vi "time_acquisition_loop.vi"(7 "Period (s)":dbl caption="周期 (s)" format="%#_13g") -> (0 "t0 (scan)":i64 caption="起始时间 (scan)", 1 "Period (scan)":i64 caption="周期 (scan)", 2 "timestamp output":timestamp caption="时间标识输出")   [LabVIEW 2015]
uses:
  globals/global_monitoring_variables.vi
  globals/global_configuration_options.vi
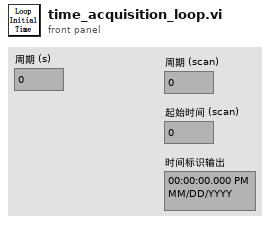
[diagram p1: front panel]
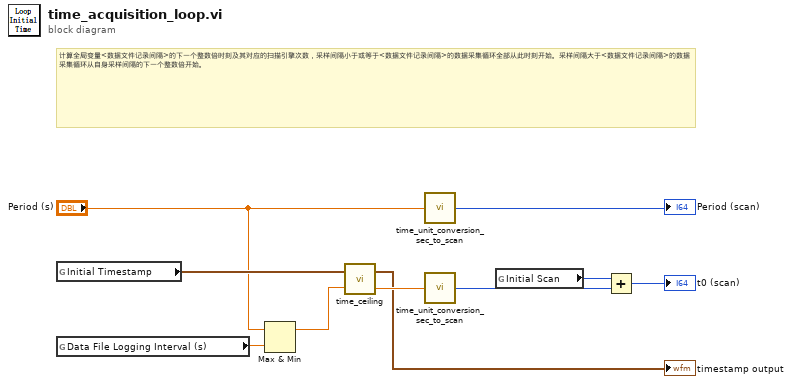
[diagram p0: block diagram]
diagram:
  # "计算全局变量<数据文件记录间隔>的下一个整数倍时刻及其对应的扫描引擎次数，采样间隔小于或等于<数据文件记录间隔>的数据采集循环全部从此时刻开始。采样间隔大于<数据文件记录间隔>的数据采集循环从自身采样间隔的下一个整数倍开始。"
  n1 = global read "global_monitoring_variables.vi" "Initial Timestamp"() -> (w10:timestamp)
  n2 = global read "global_configuration_options.vi" "Data File Logging Interval (s)"() -> (w3:dbl)
  n3 = Max & Min(x="Period (s)", y=w3) -> (max(x,y)=w2:dbl)  [unwired: 1 out]
  n4 = call "time_ceiling.vi"("base (s)"=w2, "timestamp input"=w10) -> ("time diff (s)"=w7:dbl, "timestamp output"=→"timestamp output":timestamp)
  n5 = call "time_unit_conversion_sec_to_scan.vi"("time duration (s)"="Period (s)") -> ("time duration (scan)"=→"Period (scan)":i64)
  n6 = call "time_unit_conversion_sec_to_scan.vi"("time duration (s)"=w7) -> ("time duration (scan)"=w6:i64)
  n7 = global read "global_monitoring_variables.vi" "Initial Scan"() -> (w9:i64)
  n8 = Add(x=w9, y=w6) -> (x+y=→"t0 (scan)":i64)
